vi "Constants.vi"() -> ()   [LabVIEW 2012]
uses:
  MapPOS.ctl
panel:
  in  "MapPOS":T1={"Top"={"left"=208, "top"=106, "right"=218, "bottom"=116}, "CenterC"={"left"=217, "top"=189, "right"=228, "bottom"=200}, "CenterB"={"left"=217, "top"=208, "right"=228, "bottom"=219}, "CenterA"={"left"=199, "top"=208, "right"=209, "bottom"=219}, "Left"={"left"=103, "top"=199, "right"=114, "bottom"=209}, "Right"={"left"=314, "top"=199, "right"=325, "bottom"=209}}
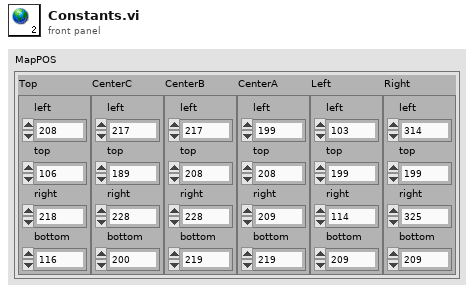
[diagram p1: front panel]
types:
  T1 = typedef "MapPOS.ctl" = cluster{"Top":cluster{"left":i16, "top":i16, "right":i16, "bottom":i16}, "CenterC":cluster{"left":i16, "top":i16, "right":i16, "bottom":i16}, "CenterB":cluster{"left":i16, "top":i16, "right":i16, "bottom":i16}, "CenterA":cluster{"left":i16, "top":i16, "right":i16, "bottom":i16}, "Left":cluster{"left":i16, "top":i16, "right":i16, "bottom":i16}, "Right":cluster{"left":i16, "top":i16, "right":i16, "bottom":i16}}
diagram:
